vi "Double Histogram (G) v2.vi"(8 "Error In":errorcluster, 9 "Histogram Options":T1={"Bin Size"=nan, "Min Value"=-inf, "Max Value"=inf, "Filter NaN & Infinite Values"=FALSE, "Frequency Plot"=FALSE, "Align Bins"=FALSE, "Bin Location"=enum."Left", "Project Outside Values"=FALSE, "Max Histogram Size"=100000} {"Max Histogram Size" format="%.0e"}, 11 "Array":dbl[](array[numeric])) -> (0 "Error Out":errorcluster, 1 "Array Statistics":T3, 2 "Histogram":dbl[](array[numeric]), 3 "Axis":dbl[](array[numeric]), 4 "Actual Bin Size":dbl)   [LabVIEW 2019]
doc: "If Min or Max are not provided, they are set to the Array Min or Max.\nIf one of the bounds is infinite, the histogram is not computed.\nIf Bin Size is not provided, or has a bogus value (< or = 0, Inf), Sturge's rule is used."
uses:
  Arrays/Array Statistics.ctl
  Histograms/Linear Histogram Options.ctl
  Histograms/Histogram Bin Position.ctl
  929807a6-00f9-4258-af09-20dfd637e3ca.vi/021b2fa1-60c1-478e-a41e-827a580c90b5.vi
  <vilib>/Utility/error.llb/Error Cluster From Error Code.vi
  <vilib>/ErrorRing/Error Ring.xnode
  <vilib>/Analysis/NI_AALBase.lvlib
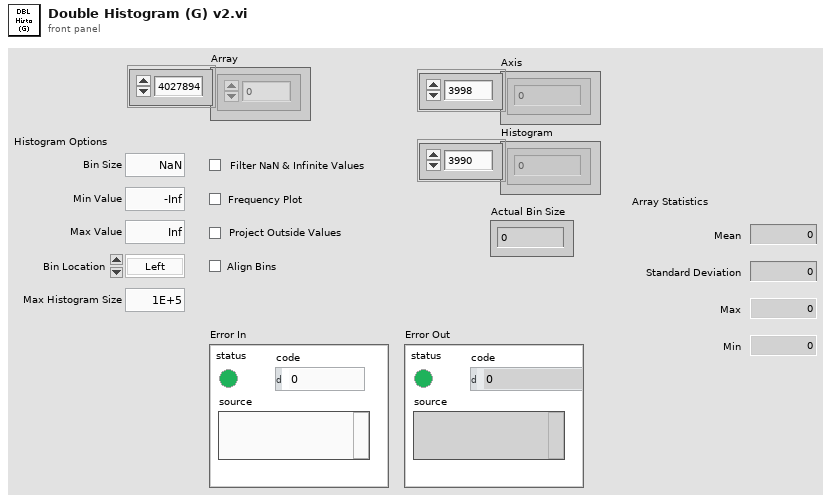
[diagram p1: front panel]
types:
  T1 = typedef "Linear Histogram Options.ctl" = cluster{"Bin Size":dbl, "Min Value":dbl, "Max Value":dbl, "Filter NaN & Infinite Values":bool, "Frequency Plot":bool, "Align Bins":bool, "Bin Location":T2, "Project Outside Values":bool, "Max Histogram Size":i32}
  T2 = typedef "Histogram Bin Position.ctl" = enum16{"Left", "Center", "Right"}
  T3 = typedef "Array Statistics.ctl" = cluster{"Mean":dbl, "Standard Deviation":dbl, "Max":dbl, "Min":dbl}
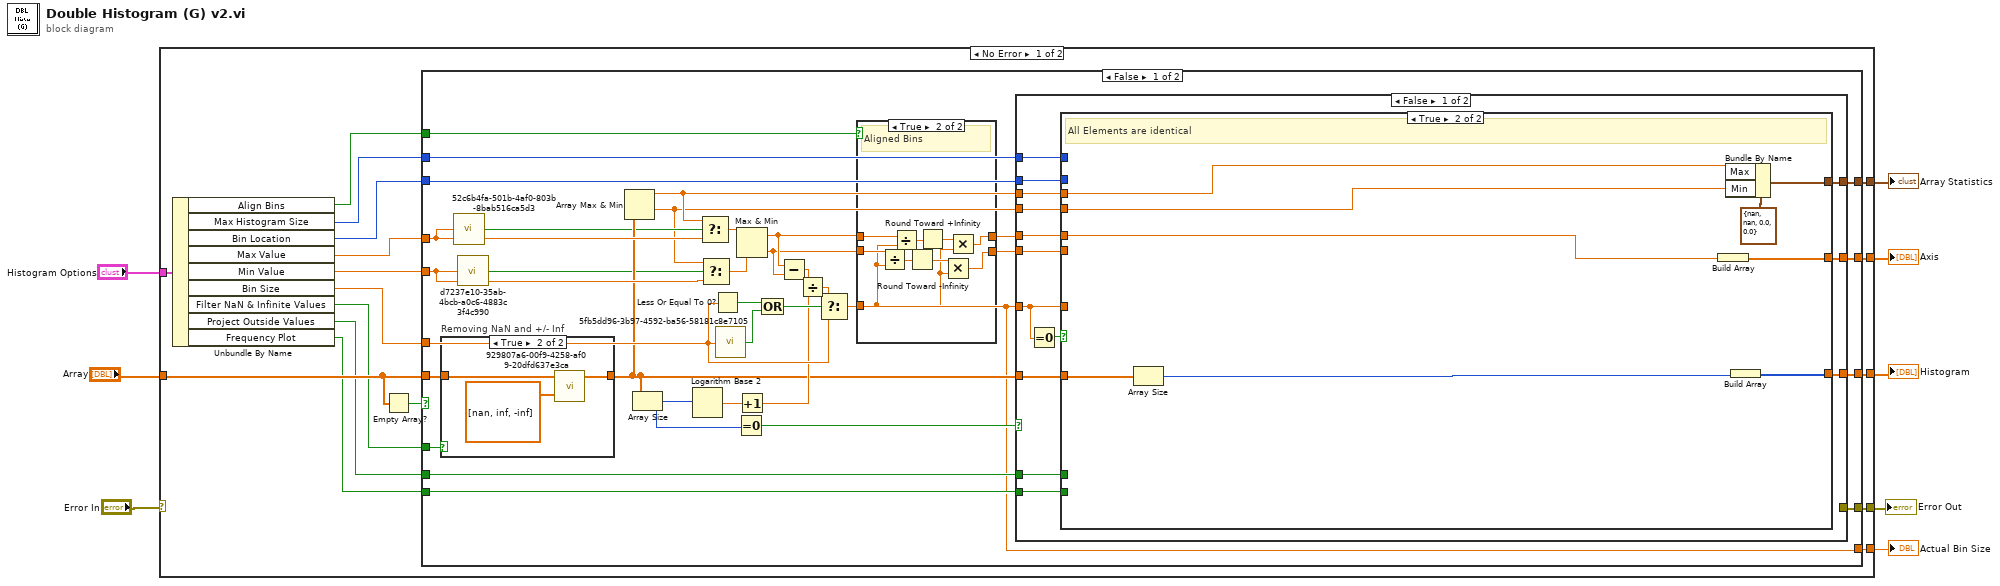
[diagram p0: block diagram]
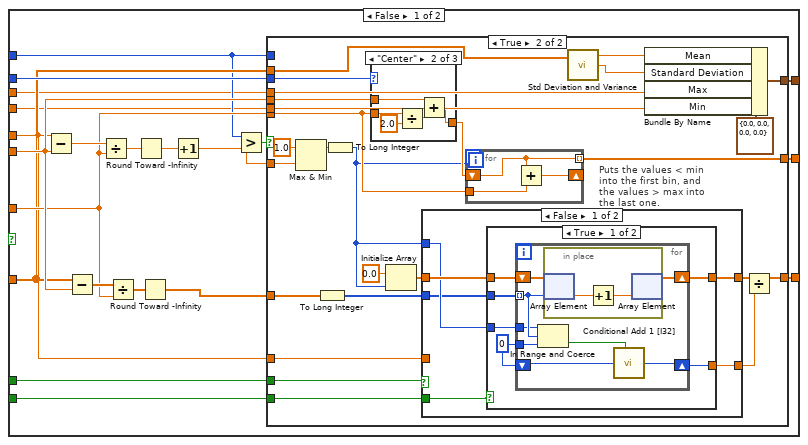
[diagram p3: hidden frame]
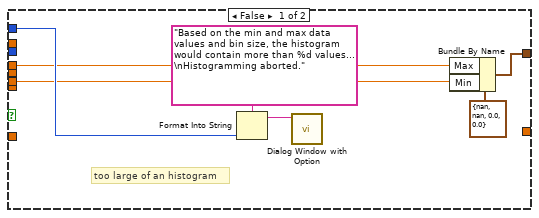
[diagram p4: hidden frame]
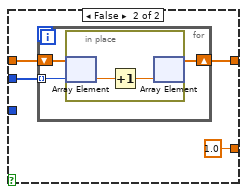
[diagram p5: hidden frame]
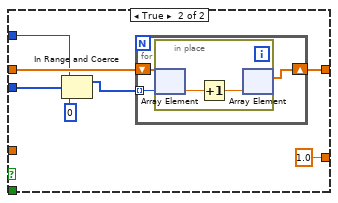
[diagram p6: hidden frame]
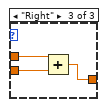
[diagram p8: hidden frame]
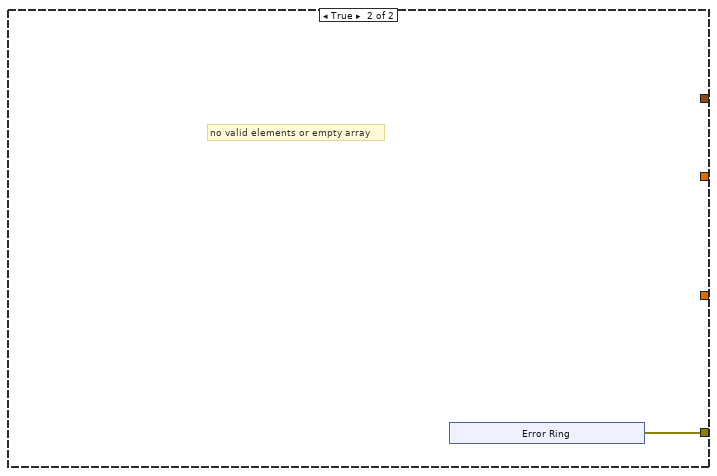
[diagram p9: hidden frame]
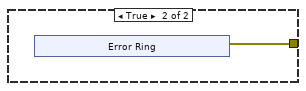
[diagram p11: hidden frame]
diagram:
  n1 = case shown="No Error" "Error In" {
    selector: "Error In" -> [_ w218]
    tunnel: [w25 _] -> w8
    tunnel: [w24 _] -> w7
    tunnel: "Array" -> [w23 _]
    tunnel: [w21 _] -> w5
    tunnel: [w20 _] -> w4
    tunnel: "Histogram Options" -> [w19 _]
    tunnel: [w9 w218] -> w1
    frame No Error {
      n2 = Unbundle By Name(w19) -> ("Align Bins"=w18:bool, "Max Histogram Size"=w17:i32, "Bin Location"=w13:T2, "Max Value"=w16:dbl, "Min Value"=w15:dbl, "Bin Size"=w14:dbl, "Filter NaN & Infinite Values"=w12:bool, "Project Outside Values"=w11:bool, "Frequency Plot"=w10:bool)
      n3 = Empty Array?(array=w23) -> (empty?=w22:bool)
      n4 = case shown="False" w22 {
        tunnel: [w60 _] -> w25
        tunnel: [w59 _] -> w24
        tunnel: w15 -> [w58 _]
        tunnel: w16 -> [w57 _]
        tunnel: w14 -> [w50 _]
        tunnel: w13 -> [w47 _]
        tunnel: w11 -> [w46 _]
        tunnel: w12 -> [w44 _]
        tunnel: w17 -> [w38 _]
        tunnel: w23 -> [w37 _]
        tunnel: [w36 _] -> w21
        tunnel: w10 -> [w35 _]
        tunnel: w18 -> [w34 _]
        tunnel: [w27 _] -> w20
        tunnel: [w26 w213] -> w9
        frame False {
          n5 = case "Removing NaN and +/- Inf" shown="True" w44 {
            tunnel: w37 -> [w209 w212]
            tunnel: [w209 w211] -> w45
            frame False {
            }
            frame True {
              n6 = call "929807a6-00f9-4258-af09-20dfd637e3ca.vi"("Element(s) to Remove"=dbl[] [nan, inf, -inf], "Input Array"=w212) -> ("Output Array"=w211:dbl[])  [unwired: 1 out]
            }
          }
          n7 = call "52c6b4fa-501b-4af0-803b-8bab516ca5d3.vi"("Number"=w57) -> ("Is NaN or Inf?"=w42:bool)  [unwired: 8 in]
          n8 = call "d7237e10-35ab-4bcb-a0c6-4883c3f4c990.vi"("Number"=w58) -> ("Is NaN or Inf?"=w43:bool)  [unwired: 8 in]
          n9 = Array Max & Min(array=w45) -> (max value=w33:dbl, min value=w32:dbl)  [unwired: 2 out]
          n10 = Array Size(array=w45) -> (size(s)=w41:i32)
          n11 = Logarithm Base 2(1:w41) -> (0:w51:dbl)
          n12 = Select(t=w33, s=w42, f=w57) -> (s? t:f=w55:dbl)
          n13 = Select(t=w32, s=w43, f=w58) -> (s? t:f=w56:dbl)
          n14 = Less Or Equal To 0?(x=w50) -> (x <= 0?=w54:bool)
          n15 = call "5fb5dd96-3b97-4592-ba56-58181c8e7105.vi"("Number"=w50) -> ("Is NaN or Inf?"=w53:bool)  [unwired: 8 in]
          n16 = Equal To 0?(x=w41) -> (x = 0?=w40:bool)
          n17 = Max & Min(x=w55, y=w56) -> (max(x,y)=w31:dbl, min(x,y)=w30:dbl)
          n18 = Increment(x=w51) -> (x+1=w48:dbl)
          n19 = Compound Arithmetic op=OR(w54, w53) -> (w52:bool)
          n20 = Subtract(x=w31, y=w30) -> (x-y=w49:dbl)
          n21 = Divide(x=w49, y=w48) -> (x/y=w39:dbl)
          n22 = Select(t=w39, s=w52, f=w50) -> (s? t:f=w27:dbl)
          n23 = case shown="True" w34 {
            tunnel: w27 -> [_ w64]
            tunnel: w31 -> [w62 w67]
            tunnel: w30 -> [w61 w71]
            tunnel: [w62 w63] -> w29
            tunnel: [w61 w68] -> w28
            frame False {
            }
            frame True {
              # "Aligned Bins"
              n24 = Divide(x=w71, y=w64) -> (x/y=w70:dbl)
              n25 = Divide(x=w67, y=w64) -> (x/y=w66:dbl)
              n26 = Round Toward -Infinity(1:w70) -> (0:w69:dbl)
              n27 = Round Toward +Infinity(x=w66) -> (ceil(x): smallest int >= x=w65:dbl)
              n28 = Multiply(x=w69, y=w64) -> (x*y=w68:dbl)
              n29 = Multiply(x=w65, y=w64) -> (x*y=w63:dbl)
            }
          }
          n30 = case shown="False" w40 {
            tunnel: [w85 _] -> w60
            tunnel: w27 -> [w78 _]
            tunnel: [w84 _] -> w59
            tunnel: w45 -> [w79 _]
            tunnel: w29 -> [w80 _]
            tunnel: w28 -> [w82 _]
            tunnel: w47 -> [w83 _]
            tunnel: w46 -> [w81 _]
            tunnel: w38 -> [w76 _]
            tunnel: [w75 _] -> w36
            tunnel: w35 -> [w74 _]
            tunnel: w33 -> [w73 _]
            tunnel: w32 -> [w72 _]
            tunnel: [_ w204] -> w26
            frame False {
              n31 = Equal To 0?(x=w78) -> (x = 0?=w77:bool)
              n32 = case shown="True" w77 {
                tunnel: [w105 w203] -> w85
                tunnel: [w102 w200] -> w84
                tunnel: w83 -> [w101 _]
                tunnel: w82 -> [w100 _]
                tunnel: w78 -> [w99 _]
                tunnel: w81 -> [w97 _]
                tunnel: w80 -> [w96 w199]
                tunnel: w79 -> [w95 w202]
                tunnel: w76 -> [w94 _]
                tunnel: [w91 w198] -> w75
                tunnel: w74 -> [w90 _]
                tunnel: w73 -> [w89 w196]
                tunnel: w72 -> [w88 w195]
                frame False {
                  n33 = Subtract(x=w96, y=w100) -> (x-y=w106:dbl)
                  n34 = Subtract(x=w95, y=w100) -> (x-y=w104:dbl[])
                  n35 = Divide(x=w106, y=w99) -> (x/y=w98:dbl)
                  n36 = Divide(x=w104, y=w99) -> (x/y=w103:dbl[])
                  n37 = Round Toward -Infinity(1:w98) -> (0:w86:dbl)
                  n38 = Round Toward -Infinity(1:w103) -> (0:w87:dbl[])
                  n39 = Increment(x=w86) -> (x+1=w93:dbl)
                  n40 = Greater?(x=w94, y=w93) -> (0:w92:bool)
                  n41 = case shown="True" w92 {
                    tunnel: [_ w139] -> w105
                    tunnel: w87 -> [_ w137]
                    tunnel: [_ w122] -> w102
                    tunnel: w101 -> [_ w135]
                    tunnel: w100 -> [_ w134]
                    tunnel: w99 -> [_ w132]
                    tunnel: w97 -> [_ w131]
                    tunnel: w96 -> [_ w130]
                    tunnel: w95 -> [_ w114]
                    tunnel: w93 -> [_ w129]
                    tunnel: w94 -> [w111 _]
                    tunnel: [w107 w125] -> w91
                    tunnel: w90 -> [_ w118]
                    tunnel: w89 -> [w110 w117]
                    tunnel: w88 -> [w109 w116]
                    frame False {
                      # "too large of an histogram"
                      n42 = Format Into String(format string="Based on the min and max data values and bin size, the histogram would contain more than %d values...\nHistogramming aborted." ("message"), w111) -> (resulting string=w113:string)  [unwired: 2 in, 1 out]
                      n43 = call "Dialog Window with Option.vi"("Message"=w113) -> ()  [unwired: 8 in, 3 out]
                      n44 = Bundle By Name(cluster=T3 {"Mean"=nan, "Standard Deviation"=nan, "Max"=0.0, "Min"=0.0} ("Array Statistics"), "Max"=w110, "Min"=w109) -> (w107:T3)
                    }
                    frame True {
                      n45 = Max & Min(x=1.0, y=w129) -> (max(x,y)=w121:dbl)  [unwired: 1 out]
                      n46 = To Long Integer(number=w137) -> (32bit integer=w119:i32[])
                      n47 = To Long Integer(number=w121) -> (32bit integer=w120:i32)
                      n48 = case shown="\"Center\"" w135 {
                        tunnel: w134 -> [w183 w186 w191]
                        tunnel: [w183 w184 w190] -> w133
                        tunnel: w132 -> [_ w188 w189]
                        frame "Left", Default {
                        }
                        frame "Center" {
                          n49 = Divide(x=w188, y=2.0) -> (x/y=w185:dbl)
                          n50 = Add(x=w186, y=w185) -> (x+y=w184:dbl)
                        }
                        frame "Right" {
                          n51 = Add(x=w191, y=w189) -> (x+y=w190:dbl)
                        }
                      }
                      n52 = Initialize Array(0.0 ("element"), w120) -> (w136:dbl[])
                      n53 = case "Puts the values < min into the first bin, and the values > max into the last one." shown="False" w131 {
                        tunnel: w119 -> [w140 w174]
                        tunnel: w136 -> [w145 w177]
                        tunnel: [w144 w176] -> w124
                        tunnel: w130 -> [_ _]
                        tunnel: w120 -> [w143 w173]
                        tunnel: [w142 1.0 ("lower limit")] -> w123
                        tunnel: w118 -> [w141 _]
                        frame False {
                          n54 = case shown="True" w141 {
                            tunnel: w145 -> [w151 w165]
                            tunnel: [w150 w164] -> w144
                            tunnel: w140 -> [w149 w163]
                            tunnel: w143 -> [w148 _]
                            tunnel: [w146 1.0 ("lower limit")] -> w142
                            frame True {
                              w147 = 0 ("lower limit")
                              n55 = for {
                                tunnel: w149 -> [w157] mode=indexing
                                shift-right: [w158] -> w150
                                shift-left: w151 -> [w159]
                                tunnel: w147 -> [w156]
                                tunnel: w148 -> [w155]
                                shift-right: [w152] -> w146
                                shift-left: w147 -> [w153]
                                n56 = In Range and Coerce(upper limit=w155, x=w157, lower limit=w156) -> (In Range?=w154:bool)  [unwired: 1 out]
                                n57 = in-place {
                                n58 = in-place-array #1(w159, w157) -> (w161:dbl)
                                n59 = Increment(x=w161) -> (x+1=w160:dbl)
                                n60 = in-place-array #1(w160) -> (w158:dbl[])  [unwired: 1 out]
                                }
                                n61 = call "Conditional Add 1 [I32].vi"("Condition"=w154, "x"=w153) -> ("x (+1)"=w152:i32)  [unwired: 7 in]
                              }
                            }
                            frame False {
                              n62 = for {
                                tunnel: w163 -> [w166] mode=indexing
                                shift-right: [w167] -> w164
                                shift-left: w165 -> [w168]
                                n63 = in-place {
                                n64 = in-place-array #2(w168, w166) -> (w170:dbl)
                                n65 = Increment(x=w170) -> (x+1=w169:dbl)
                                n66 = in-place-array #2(w169) -> (w167:dbl[])  [unwired: 1 out]
                                }
                              }
                            }
                          }
                        }
                        frame True {
                          n67 = In Range and Coerce(upper limit=w173, x=w174, lower limit=0) -> (coerced(x)=w172:i32[])  [unwired: 1 out]
                          n68 = for {
                            shift-right: [w179] -> w176
                            shift-left: w177 -> [w180]
                            tunnel: w172 -> [w178] mode=indexing
                            n69 = in-place {
                              n70 = in-place-array #3(w180, w178) -> (w182:dbl)
                              n71 = Increment(x=w182) -> (x+1=w181:dbl)
                              n72 = in-place-array #3(w181) -> (w179:dbl[])  [unwired: 1 out]
                            }
                          }
                        }
                      }
                      n73 = for {
                        N: w120 -> [_]
                        shift-right: [w193] -> _
                        shift-left: w133 -> [w192]
                        tunnel: w132 -> [w194]
                        tunnel: [w192] -> w139 mode=indexing
                        n74 = Add(x=w192, y=w194) -> (x+y=w193:dbl)
                      }
                      n75 = call <vilib>:"Std Deviation and Variance.vi"("X"=w114) -> ("mean"=w127:dbl, "standard deviation"=w126:dbl)  [unwired: 1 in, 1 out]
                      n76 = Bundle By Name(cluster=T3 {"Mean"=0.0, "Standard Deviation"=0.0, "Max"=0.0, "Min"=0.0} ("Array Statistics"), "Mean"=w127, "Standard Deviation"=w126, "Max"=w117, "Min"=w116) -> (w125:T3)
                      n77 = Divide(x=w124, y=w123) -> (x/y=w122:dbl[])
                    }
                  }
                }
                frame True {
                  # "All Elements are identical"
                  n78 = Array Size(array=w202) -> (size(s)=w201:i32)
                  n79 = Build Array(w199) -> (w203:dbl[])
                  n80 = Bundle By Name(cluster=T3 {"Mean"=nan, "Standard Deviation"=nan, "Max"=0.0, "Min"=0.0} ("Array Statistics"), "Max"=w196, "Min"=w195) -> (w198:T3)
                  n81 = Build Array(w201) -> (w200:i32[])
                }
              }
            }
            frame True {
              # "no valid elements or empty array"
              n82 = xnode "Error Ring"() -> ("error out"=w204:errorcluster)
            }
          }
        }
        frame True {
          n83 = xnode "Error Ring"() -> ("error out"=w213:errorcluster)
        }
      }
    }
    frame Error {
    }
  }
  "Histogram" <- w7
  "Axis" <- w8
  "Array Statistics" <- w5
  "Actual Bin Size" <- w4
  "Error Out" <- w1
